vi "HTTP Request.vi"(0 "REST Client in":refnum<class "REST Client_JKI.lvclass">, 1 "Request body":string, 2 "Multipart Post data":T1[](array[typedef]), 5 "Method":T2, 9 "Path":string, 11 "error in (no error)":errorcluster, 12 "request specific headers":T3[](array[typedef]), 13 "timeout (0 = Use Default)":i32) -> (3 "Status Code":u16, 4 "REST Client out":refnum<class "REST Client_JKI.lvclass">, 6 "Response Headers out":refnum<class "Response Headers.lvclass">, 10 "Response body":string, 14 "Status String":string, 15 "error out":errorcluster)   [LabVIEW 2018, in "REST Client.lvlib" / "REST Client_JKI.lvclass"]
uses:
  REST Client_JKI.lvclass
  C:/Viviota/Projects/R&D/LabVIEW_HTTP_REST_Client/source/classes/REST Client/REST Client.lvclass
  Response Headers/Response Headers.lvclass
  REST Client/HTTP Header.ctl
  REST Client/HTTP Methods.ctl
  <vilib>/httpClient/MultipartData.ctl
  <vilib>/httpClient/POSTBuffer.vi
  <vilib>/httpClient/LabVIEWHTTPClient.lvlib
  REST Client/REST Client.lvclass
panel:
  # "Copyright © 2014 JKI All rights reserved.\n\nAuthor: Tomi Maila <tomi.maila@jki.net>\n\nThis library is provided \"AS IS\" ,WITHOUT WARRANTIES OR \nCONDITIONS OF ANY KIND, either express or implied.\n\nJKI -- jki.net"
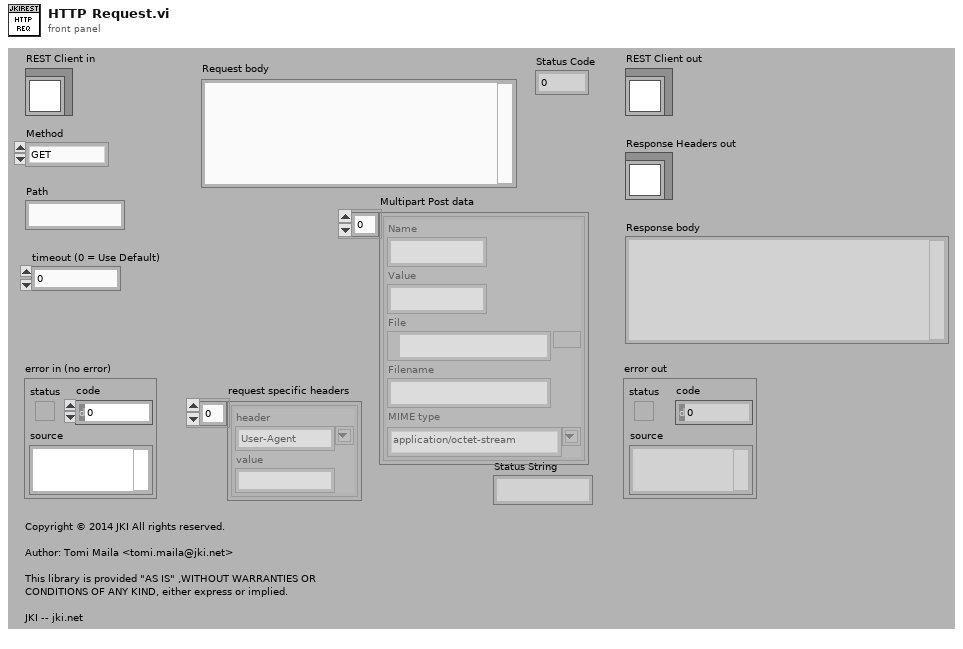
[diagram p1: front panel]
types:
  T1 = typedef "LabVIEWHTTPClient.lvlib/MultipartData.ctl" = cluster{"Name":string, "Value":string, "File":path, "Filename":string, "MIME type":string}
  T2 = typedef "REST Client.lvlib/REST Client.lvclass/HTTP Methods.ctl" = enum16{"GET", "HEAD", "POST", "PUT", "DELETE"}
  T3 = typedef "REST Client.lvlib/REST Client.lvclass/HTTP Header.ctl" = cluster{"header":string, "value":string}
  T4 = typedef "LabVIEWHTTPClient.lvlib/ClientHandle.ctl" = refnum<k1>
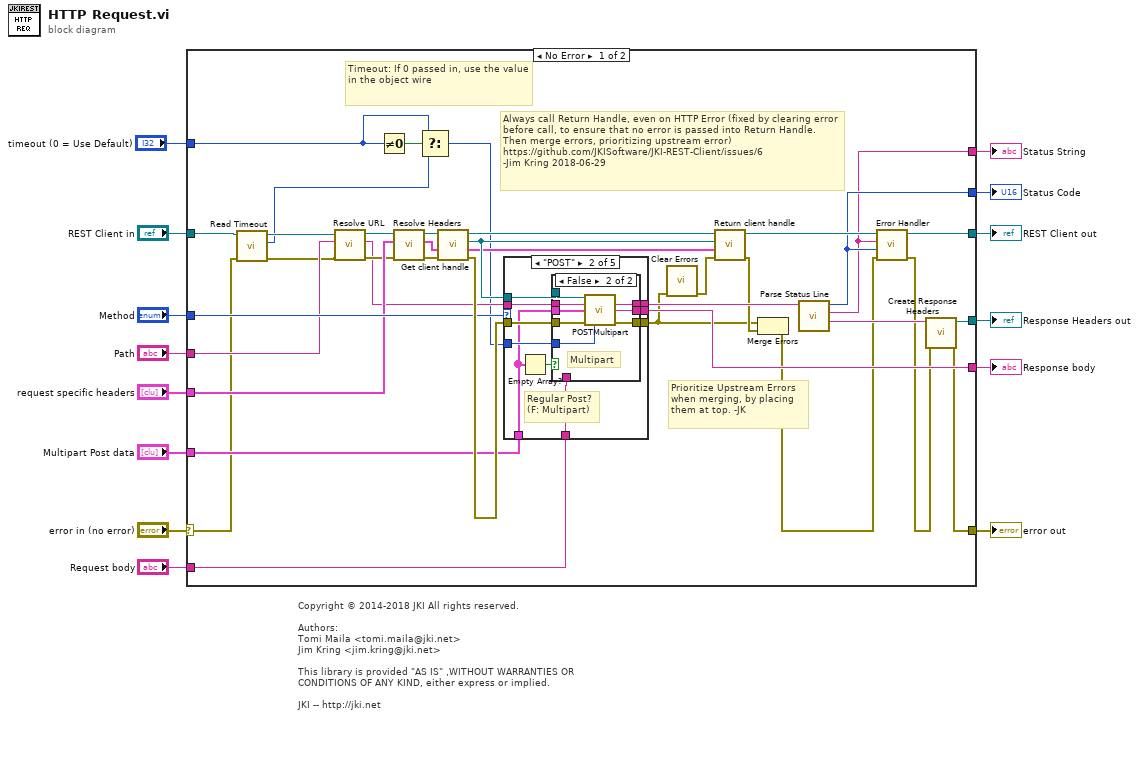
[diagram p0: block diagram]
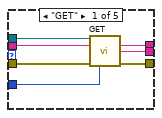
[diagram p2: hidden frame]
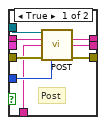
[diagram p3: hidden frame]
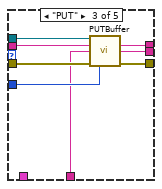
[diagram p4: hidden frame]
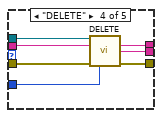
[diagram p5: hidden frame]
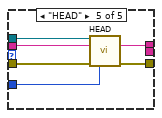
[diagram p6: hidden frame]
diagram:
  # "Copyright © 2014-2018 JKI All rights reserved.\n\nAuthors:\nTomi Maila <tomi.maila@jki.net>\nJim Kring <jim.kring@jki.net>\n\nThis library is provided \"AS IS\" ,WITHOUT WARRANTIES OR \nCONDITIONS OF ANY KIND, either express or implied.\n\nJKI -- http://jki.net"
  n1 = case shown="No Error" "error in (no error)" {
    selector: "error in (no error)" -> [w18 w107]
    tunnel: [w28 w107] -> w13
    tunnel: [w44 w106] -> w11
    tunnel: "REST Client in" -> [w19 w106]
    tunnel: "Method" -> [w43 _]
    tunnel: "Path" -> [w36 _]
    tunnel: "Request body" -> [w50 _]
    tunnel: [w32 _] -> w8
    tunnel: [w30 _] -> w3
    tunnel: [w34 _] -> w7
    tunnel: "request specific headers" -> [w41 _]
    tunnel: [w33 _] -> w4
    tunnel: "Multipart Post data" -> [w27 _]
    tunnel: "timeout (0 = Use Default)" -> [w21 _]
    frame No Error {
      # "Timeout: If 0 passed in, use the value in the object wire"
      # "Prioritize Upstream Errors when merging, by placing them at top. -JK"
      # "Always call Return Handle, even on HTTP Error (fixed by clearing error before call, to ensure that no error is passed into Return Handle. Then merge errors, prioritizing upstream error)\nhttps://github.com/JKISoftware/JKI-REST-Client/issues/6\n-Jim Kring 2018-06-29"
      n2 = call-dynamic "Read Timeout.vi"("error in (no error)"=w18, "REST Client in"=w19) -> ("error out"=w17:errorcluster, "Timeout"=w15:i32, "REST Client out"=w16:refnum<class "REST Client_JKI.lvclass">)  [unwired: 7 in]
      n3 = call "Resolve URL.vi"("error in (no error)"=w17, "Path"=w36, "REST Client in"=w16) -> ("error out"=w37:errorcluster, "Resolved URL"=w35:string, "REST Client out"=w38:refnum<class "REST Client_JKI.lvclass">)  [unwired: 6 in]
      n4 = Not Equal To 0?(x=w21) -> (x != 0?=w22:bool)
      n5 = call "Resolve Headers.vi"("error in (no error)"=w37, "headers in"=w41, "REST Client in"=w38) -> ("error out"=w39:errorcluster, "headers out"=w40:T3[], "REST Client out"=w42:refnum<class "REST Client_JKI.lvclass">)  [unwired: 6 in]
      n6 = Select(t=w21, s=w22, f=w15) -> (s? t:f=w20:i32)
      n7 = call "Get client handle.vi"("error in (no error)"=w39, "headers"=w40, "REST Client in"=w42) -> ("error out"=w49:errorcluster, "headers out"=w46:T3[], "Client Handle"=w47:T4, "REST Client out"=w48:refnum<class "REST Client_JKI.lvclass">)  [unwired: 5 in]
      n8 = case shown="\"POST\"" w43 {
        tunnel: w35 -> [w58 w68 w92 w99 w105]
        tunnel: w20 -> [w57 w67 w91 w98 w104]
        tunnel: w49 -> [w56 w66 w90 w97 w103]
        tunnel: [w55 w65 w89 w96 w102] -> w51
        tunnel: [w54 w64 w88 w95 _] -> w34
        tunnel: [w53 w63 w87 w94 w101] -> w24
        tunnel: w47 -> [w52 w62 w86 w93 w100]
        tunnel: w50 -> [_ w61 w85 _ _]
        tunnel: w27 -> [_ w59 _ _ _]
        frame "GET" {
          n9 = call <vilib>:"GET.vi"("client handle"=w52, "url"=w58, "error in (no error)"=w56, "timeout (10000)"=w57) -> ("headers"=w55:string, "body"=w54:string, "error out"=w53:errorcluster)  [unwired: 8 in, 1 out]
        }
        frame "POST" {
          # "Regular Post?\n(F: Multipart)"
          n10 = Empty Array?(array=w59) -> (empty?=w60:bool)
          n11 = case shown="False" w60 {
            tunnel: w68 -> [w76 w84]
            tunnel: w67 -> [w75 w83]
            tunnel: w66 -> [w74 w82]
            tunnel: [w73 w81] -> w65
            tunnel: [w72 w80] -> w64
            tunnel: [w71 w79] -> w63
            tunnel: w62 -> [w70 w78]
            tunnel: w61 -> [w69 _]
            tunnel: w59 -> [_ w77]
            frame True {
              # "Post"
              n12 = call-poly <vilib>:"POST.vi"("client handle"=w70, "url"=w76, "buffer"=w69, "error in (no error)"=w74, "timeout (10000)"=w75) -> ("headers"=w73:string, "body"=w72:string, "error out"=w71:errorcluster)  [unwired: 7 in, 1 out]
            }
            frame False {
              # "Multipart"
              n13 = call <vilib>:"POSTMultipart.vi"("client handle"=w78, "url"=w84, "data"=w77, "error in (no error)"=w82, "timeout (10000)"=w83) -> ("headers"=w81:string, "body"=w80:string, "error out"=w79:errorcluster)  [unwired: 7 in, 1 out]
            }
          }
        }
        frame "PUT" {
          n14 = call <vilib>:"PUTBuffer.vi"("client handle"=w86, "url"=w92, "buffer"=w85, "error in (no error)"=w90, "timeout (10000)"=w91) -> ("headers"=w89:string, "body"=w88:string, "error out"=w87:errorcluster)  [unwired: 7 in, 1 out]
        }
        frame "DELETE" {
          n15 = call <vilib>:"DELETE.vi"("client handle"=w93, "url"=w99, "error in (no error)"=w97, "timeout (10000)"=w98) -> ("headers"=w96:string, "body"=w95:string, "error out"=w94:errorcluster)  [unwired: 8 in, 1 out]
        }
        frame "HEAD" {
          n16 = call <vilib>:"HEAD.vi"("client handle"=w100, "url"=w105, "error in (no error)"=w103, "timeout (10000)"=w104) -> ("headers"=w102:string, "error out"=w101:errorcluster)  [unwired: 9 in, 1 out]
        }
      }
      n17 = call <vilib>:"Clear Errors.vi"("error in (no error)"=w24) -> ("error out"=w23:errorcluster)  [unwired: 5 in, 1 out]
      n18 = call "Return client handle.vi"("error in (no error)"=w23, "headers"=w46, "Client Handle"=w47, "REST Client in"=w48) -> ("error out"=w26:errorcluster, "REST Client out"=w45:refnum<class "REST Client_JKI.lvclass">)  [unwired: 6 in]
      n19 = Merge Errors(w24, w26) -> (w25:errorcluster)
      n20 = call "Parse Status Line.vi"("Headers w/ status line"=w51) -> ("HTTP Headers"=w31:string, "Status String"=w32:string, "Status Code"=w33:u16)  [unwired: 6 in, 2 out]
      n21 = call-dynamic "Error Handler.vi"("error in (no error)"=w25, "Status Code"=w33, "Status String"=w32, "REST Client in"=w45) -> ("error out"=w29:errorcluster, "REST Client out"=w44:refnum<class "REST Client_JKI.lvclass">)  [unwired: 6 in]
      n22 = call "Create Response Headers.vi"("error in (no error)"=w29, "Response Headers"=w31) -> ("error out"=w28:errorcluster, "Response Headers out"=w30:refnum<class "Response Headers.lvclass">)  [unwired: 8 in]
    }
    frame Error {
    }
  }
  "error out" <- w13
  "REST Client out" <- w11
  "Status Code" <- w4
  "Status String" <- w8
  "Response Headers out" <- w3
  "Response body" <- w7
